vi "textParse.vi"(8 "error in (no error)":errorcluster, 10 "file name":string, 11 "base path":path=path "C:/Users/bryan.lee/Desktop/Specification sheets") -> (0 "error out":errorcluster, 2 "all rows":string[][](array[string]), 3 "appended path":path)   [LabVIEW 2018]
uses:
  <vilib>/Utility/file.llb/Read Delimited Spreadsheet (string).vi
panel:
  out "LED Frequency Max":string
  out "LED Frequency Min":string
  out "LED Frequency (Charge)":string
  out "LED Frequency (Limit)":string
  out "LED Frequency (Foldback)":string
  out "HV Bus Voltage(@10% PWM)":string
  out "HV Bus Tol. Min":string
  out "HV Bus Tol. Max":string
  out "Speed Pot Voltage Low(@85% PWM)":string
  out "Speed Pot Voltage Mid(@85% PWM)":string
  out "Speed Pot Voltage High(@85% PWM)":string
  out "Speed Pot Voltage Tol. Min":string
  out "Speed Pot Voltage Tol. Max":string
  out "Ircomp(@70% PWM)":string
  out "Ircomp Voltage Tol. Min":string
  out "Ircomp Voltage Tol. Max":string
  out "Current Limit(@45% PWM)":string
  out "Sense Voltage Tol. Max":string
  out "Sense Voltage Tol. Min":string
  out "Sense Voltage":string
  out "Allowable Power Interuption":string
  out "Voltage FET Driver Tol. Max":string
  out "Voltage FET Driver Tol. Min":string
  out "Voltage FET Driver":string
  out "Voltage Micro Tol. Max":string
  out "Voltage Micro Tol. Min":string
  out "Voltage Micro":string
  out "Rated Output Current Tol. Max":string
  out "Rated Output Current Tol. Min":string
  out "Rated Output Current":string
  out "Ripple/Noise Tol. Max":string
  out "Ripple/Noise Tol. Min":string
  out "Ripple/Noise":string
  out "Voltage Output Tol. Max":string
  out "Voltage  Output Tol. Min":string
  out "Voltage Output":string
  out "Max Input Current":string
  out "Input Current":string
  out "Input Voltage Tol. Max":string
  out "Input Voltage Tol. Min":string
  out "Input Voltage":string
  out "Vendor Number":string
  out "Vendor Name":string
  out "Firmware":string
  out "Part Number":string
  out "Part Name":string
  # "Global variables"
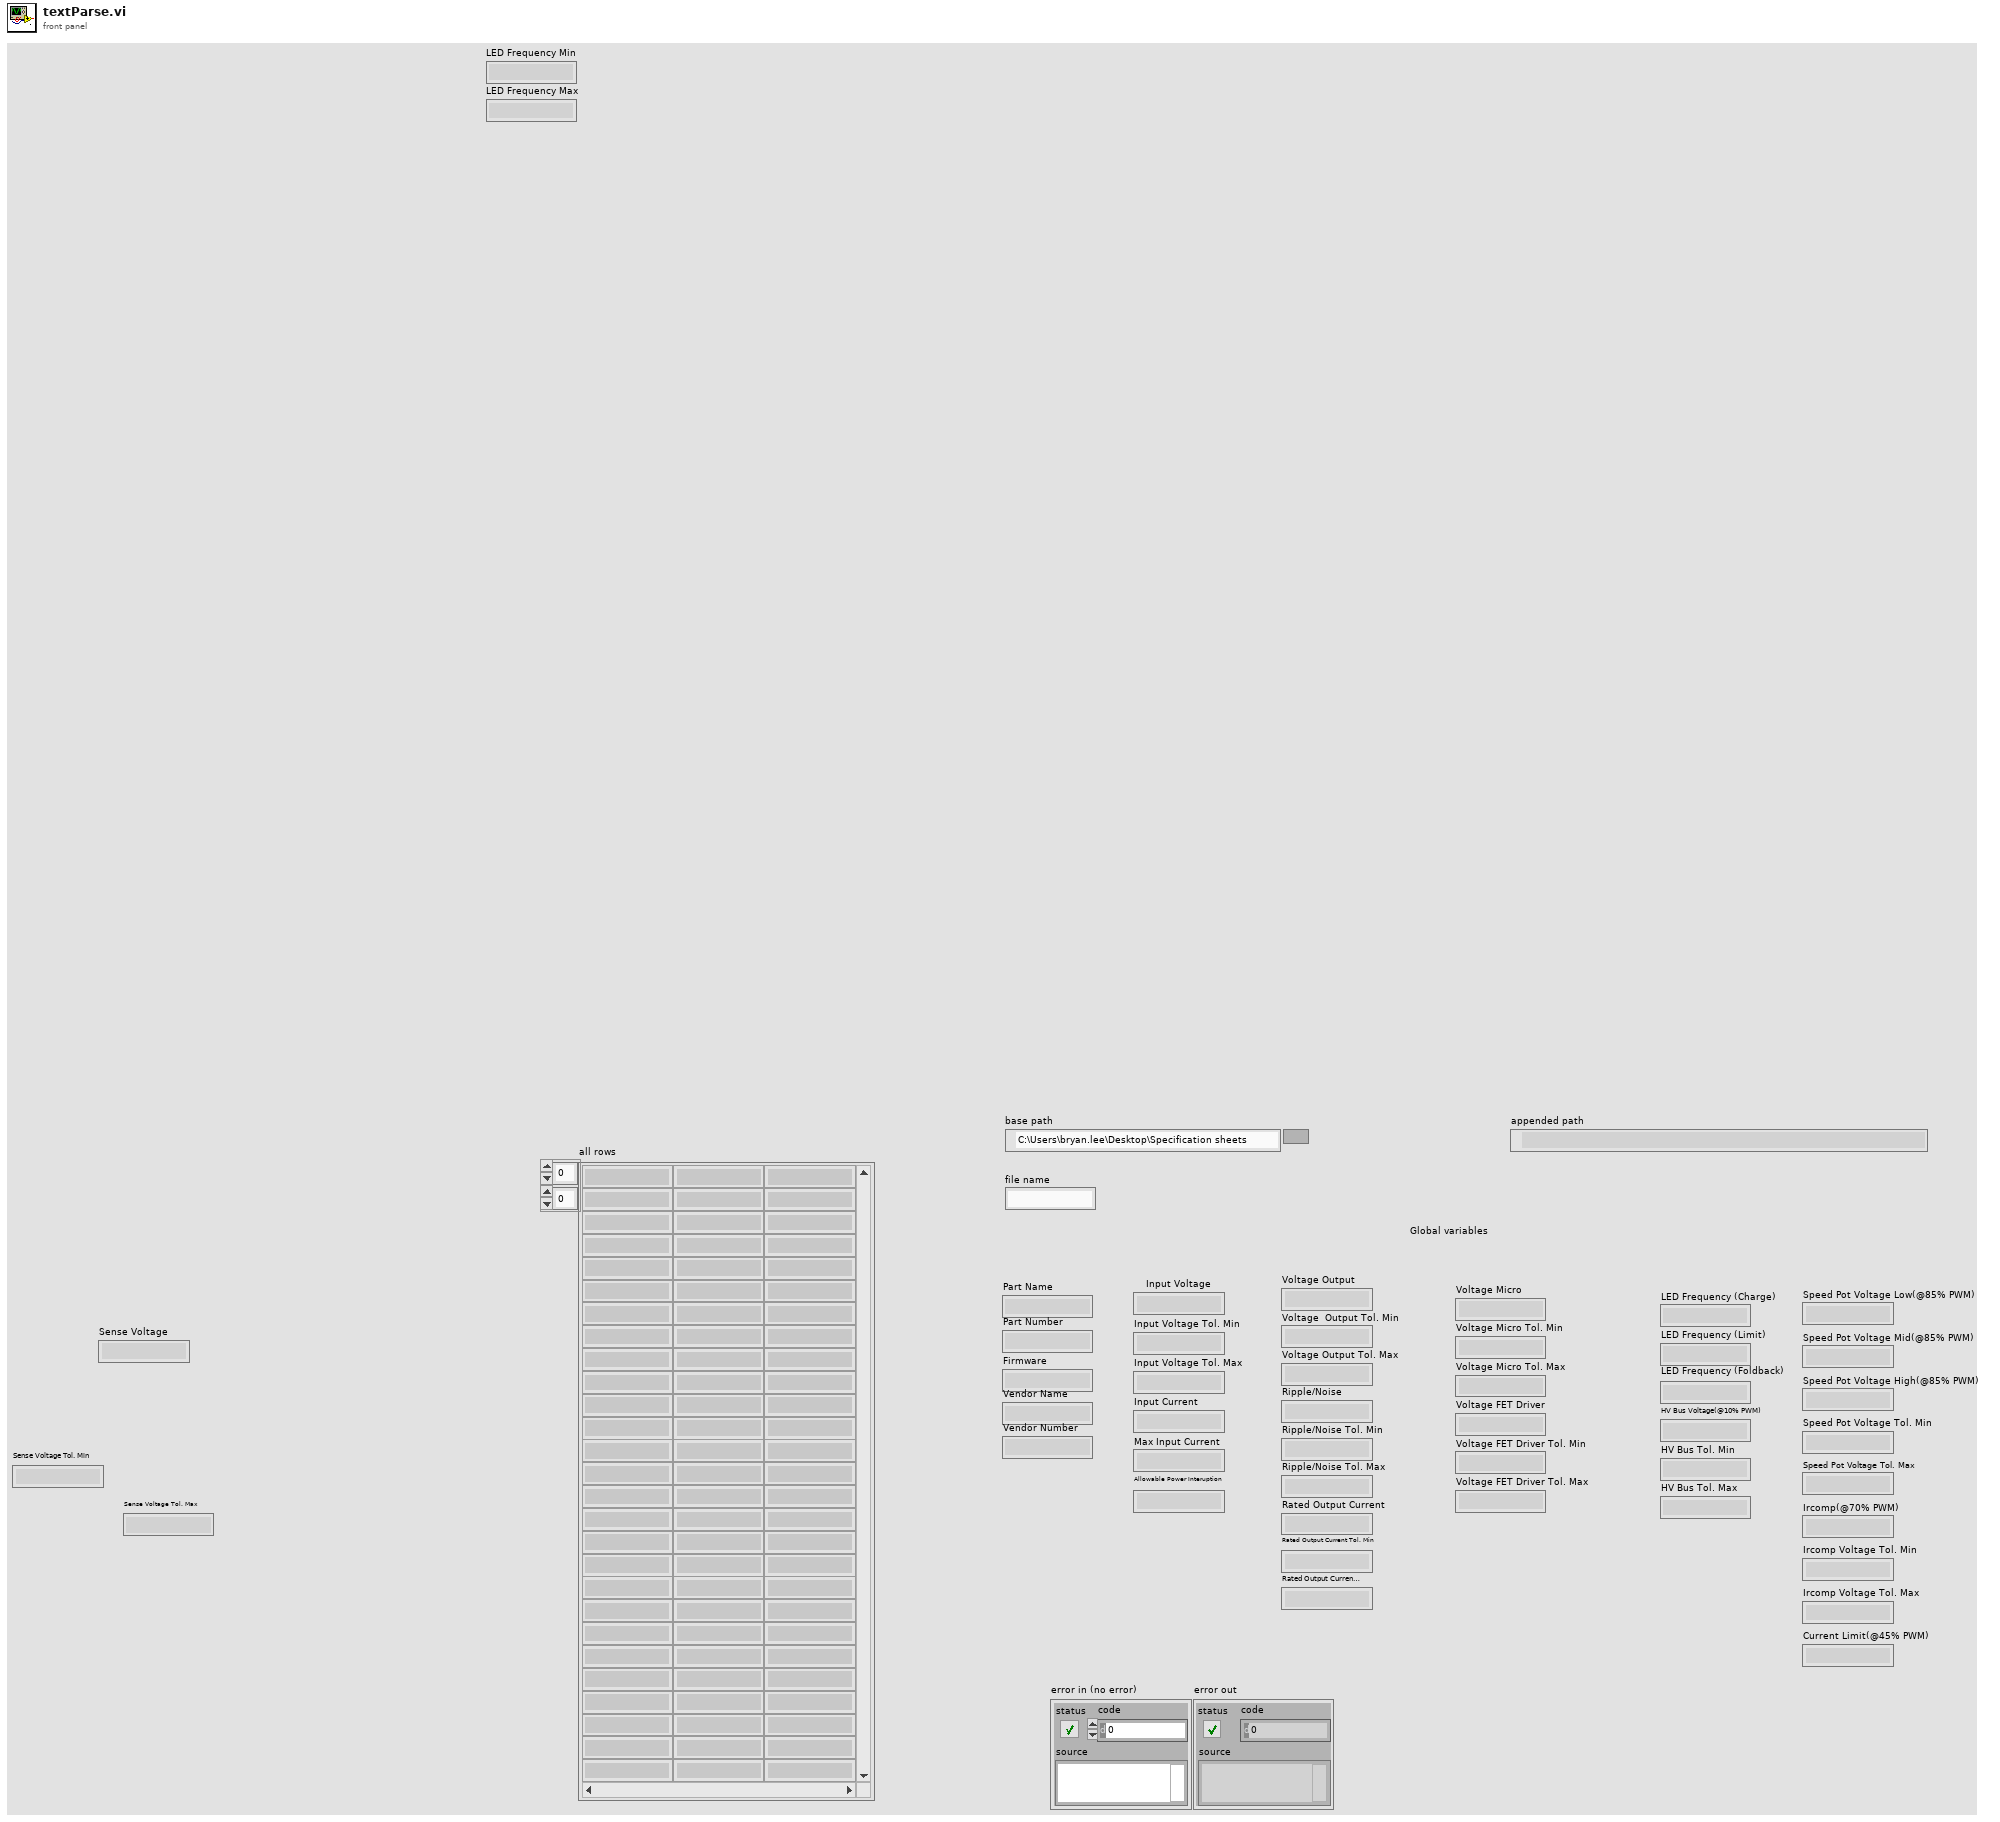
[diagram p1: front panel]
types:
  T1 = enum16{"Main", "In Primary", "Secondary", "Out Primary", "Motor Drive", ""}
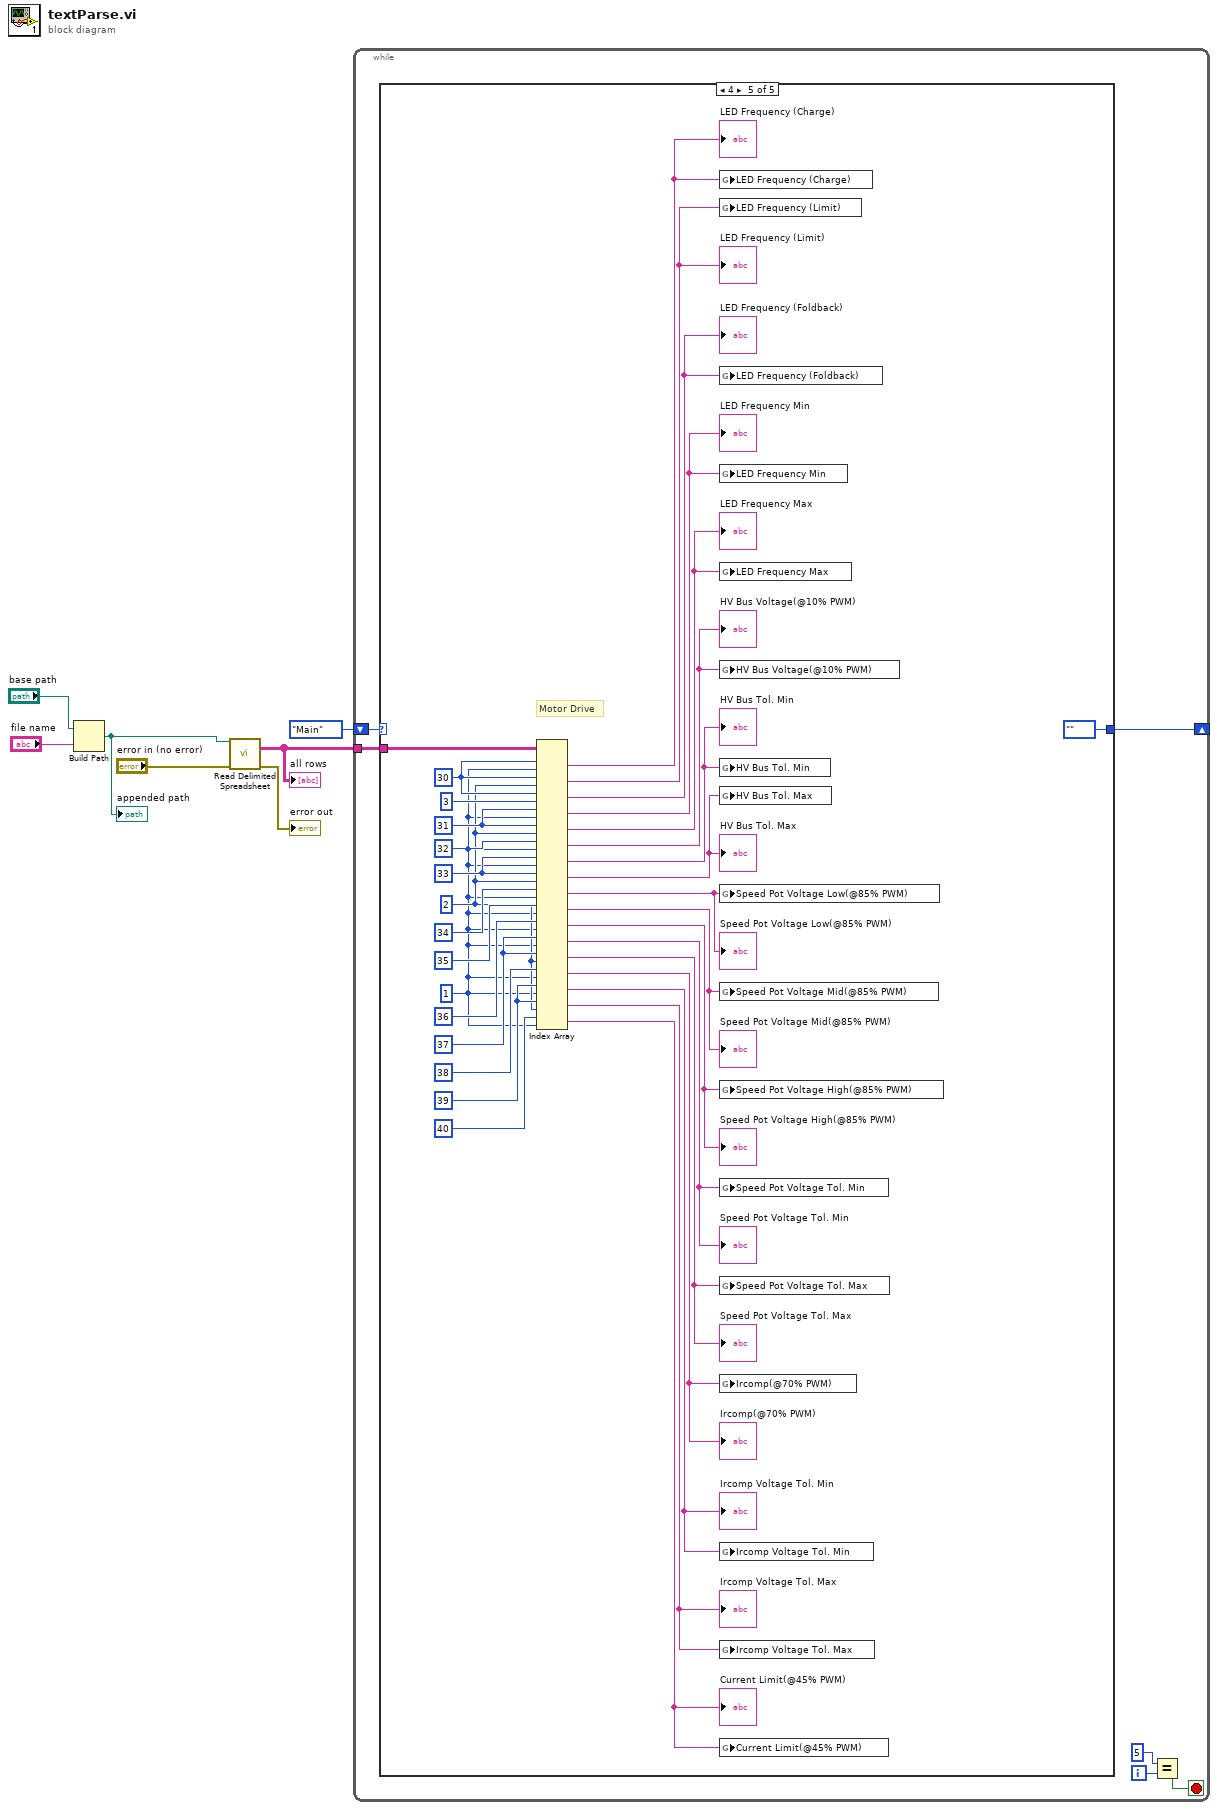
[diagram p0: block diagram]
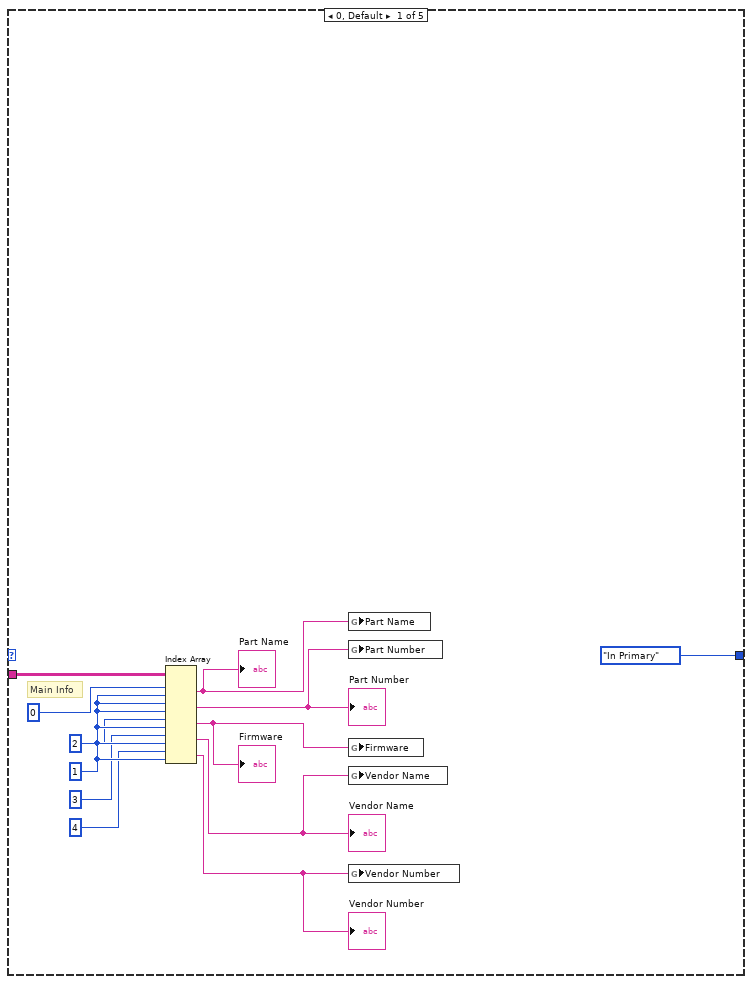
[diagram p2: hidden frame]
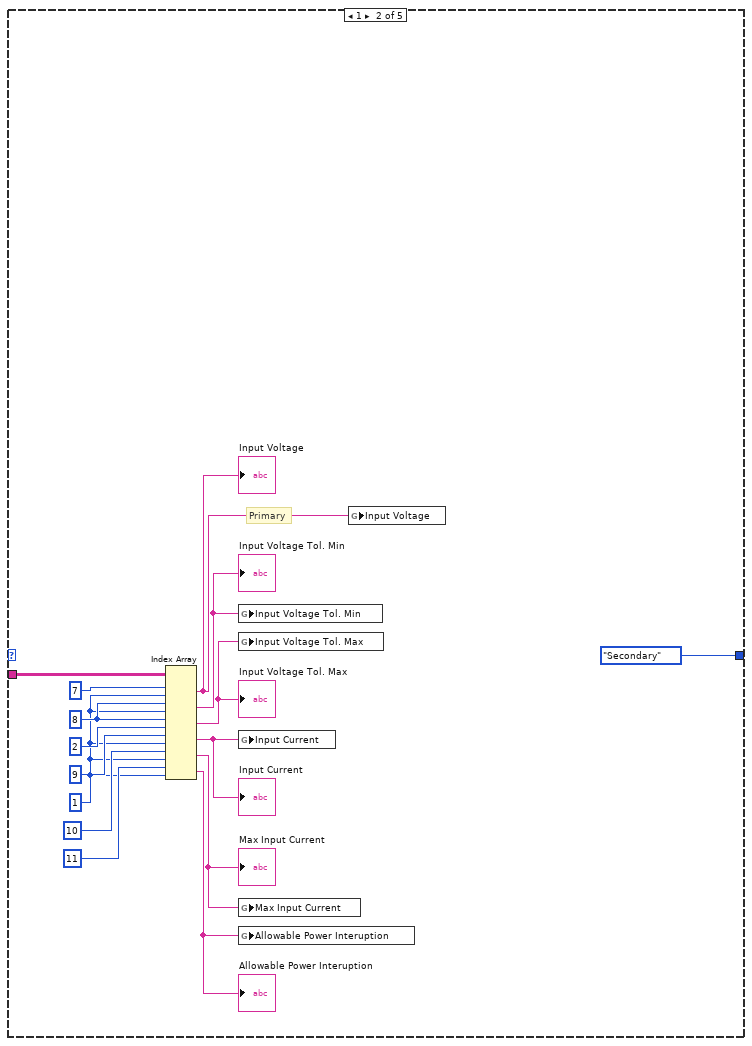
[diagram p3: hidden frame]
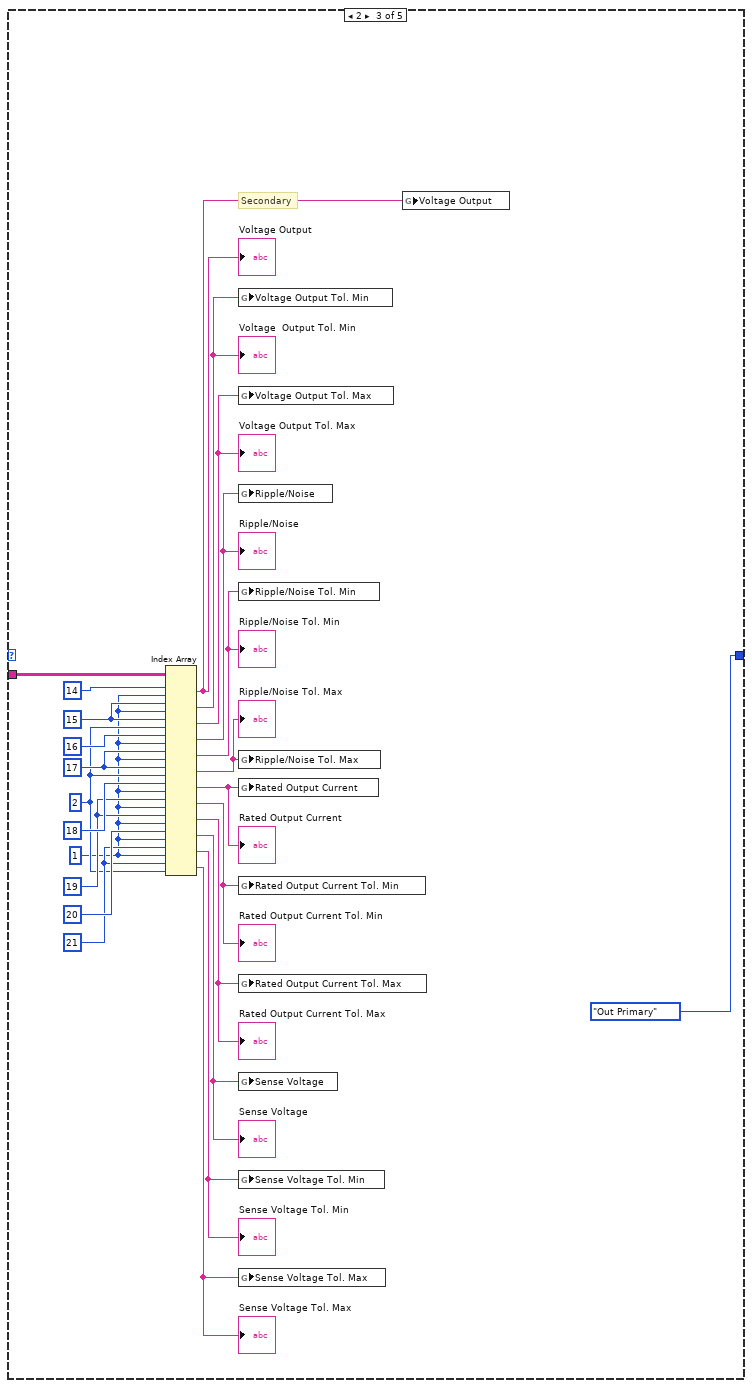
[diagram p4: hidden frame]
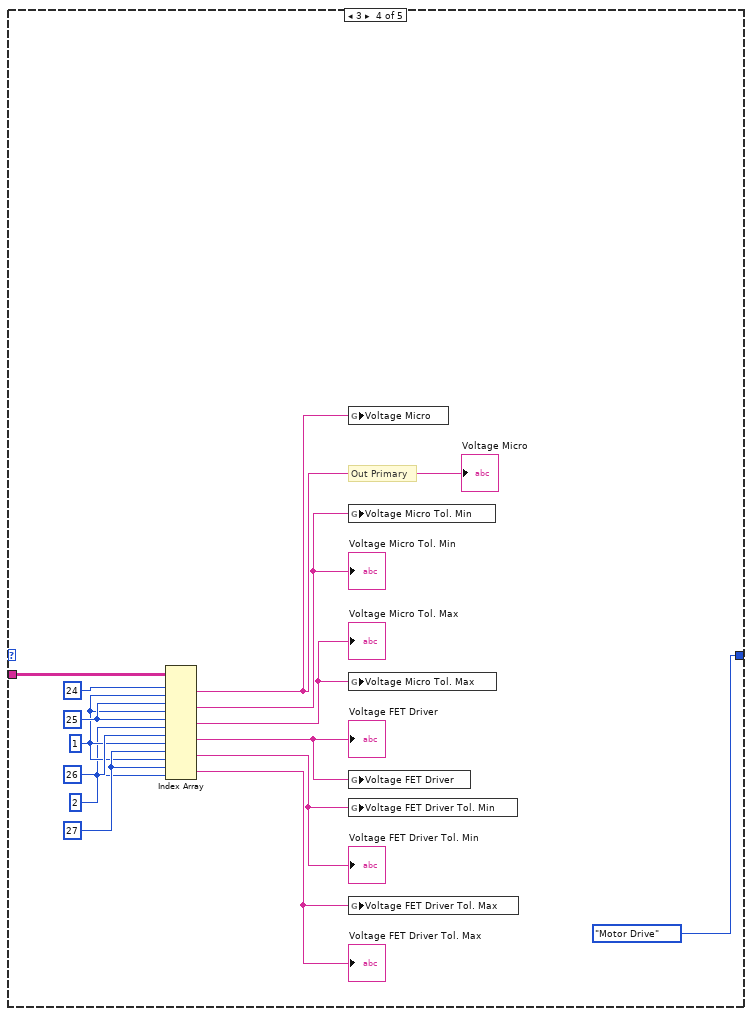
[diagram p5: hidden frame]
diagram:
  n1 = Build Path(base path="base path", name or relative path="file name") -> (appended path=w5:path)
  "appended path" <- w5
  n2 = call-poly <vilib>:"Read Delimited Spreadsheet.vi"("file path (dialog if empty)"=w5, "error in (no error)"="error in (no error)") -> ("all rows"=w2:string[][], "error out"=→"error out":errorcluster)  [unwired: 8 in, 4 out]
  "all rows" <- w2
  n3 = while {
    shift-right: [w12] -> _
    shift-left: T1."Main" -> [w8]
    tunnel: w2 -> [w9]
    i -> [w11]
    stop <- w13 stop-if-true
    n4 = case shown="4" w8 {
      tunnel: w9 -> [w15 w29 w49 w68 w110]
      tunnel: [T1."In Primary" T1."Secondary" T1."Out Primary" T1."Motor Drive" enum16{""}.""] -> w12
      frame 0, Default {
        w19 = 1
        # "Main Info"
        n5 = Index Array(array=w15, index (row) #1=0 ("index (row)"), index (col) #1=w19, index (row) #2=w19, index (col) #2=w19, index (row) #3=2 ("index (row)"), index (col) #3=w19, index (row) #4=3 ("disabled index (row)"), index (col) #4=w19, index (row) #5=4 ("disabled index (row)"), index (col) #5=w19) -> (element #1=w21:string, element #2=w23:string, element #3=w22:string, element #4=w24:string, element #5=w25:string)
        "Part Name" <- w21
        "Part Number" <- w23
        "Firmware" <- w22
        "Vendor Name" <- w24
        "Vendor Number" <- w25
        n6 = global write "Global textParse.vi" "Part Name"(w21) -> ()
        n7 = global write "Global textParse.vi" "Part Number"(w23) -> ()
        n8 = global write "Global textParse.vi" "Firmware"(w22) -> ()
        n9 = global write "Global textParse.vi" "Vendor Name"(w24) -> ()
        n10 = global write "Global textParse.vi" "Vendor Number"(w25) -> ()
      }
      frame 1 {
        w33 = 8
        w27 = 1
        # "Primary"
        n11 = Index Array(array=w29, index (row) #1=7, index (col) #1=w27, index (row) #2=w33, index (col) #2=w27, index (row) #3=w33, index (col) #3=2, index (row) #4=9, index (col) #4=w27, index (row) #5=10, index (col) #5=w27, index (row) #6=11, index (col) #6=w27) -> (element #1=w35:string, element #2=w36:string, element #3=w37:string, element #4=w38:string, element #5=w39:string, element #6=w40:string)
        "Input Voltage" <- w35
        "Input Voltage Tol. Min" <- w36
        "Input Voltage Tol. Max" <- w37
        "Input Current" <- w38
        "Max Input Current" <- w39
        "Allowable Power Interuption" <- w40
        n12 = global write "Global textParse.vi" "Input Voltage Tol. Min"(w36) -> ()
        n13 = global write "Global textParse.vi" "Input Voltage Tol. Max"(w37) -> ()
        n14 = global write "Global textParse.vi" "Input Current"(w38) -> ()
        n15 = global write "Global textParse.vi" "Max Input Current"(w39) -> ()
        n16 = global write "Global textParse.vi" "Allowable Power Interuption"(w40) -> ()
        n17 = global write "Global textParse.vi" "Input Voltage"(w35) -> ()
      }
      frame 2 {
        w47 = 21 ("index (row)")
        w50 = 19 ("index (row)")
        w45 = 1
        w46 = 2
        w52 = 17 ("index (row) 15")
        w54 = 15 ("index (row) 13")
        # "Secondary"
        n18 = Index Array(array=w49, index (row) #1=14 ("index (row) 12"), index (col) #1=w45, index (row) #2=w54, index (col) #2=w45, index (row) #3=w54, index (col) #3=w46, index (row) #4=16 ("index (row) 14"), index (col) #4=w45, index (row) #5=w52, index (col) #5=w45, index (row) #6=w52, index (col) #6=w46, index (row) #7=18 ("index (row) 19"), index (col) #7=w45, index (row) #8=w50, index (col) #8=w45, index (row) #9=w50, index (col) #9=w45, index (row) #10=20 ("index (row)"), index (col) #10=w45, index (row) #11=w47, index (col) #11=w45, index (row) #12=w47, index (col) #12=w46) -> (element #1=w56:string, element #2=w57:string, element #3=w58:string, element #4=w59:string, element #5=w60:string, element #6=w61:string, element #7=w62:string, element #8=w63:string, element #9=w64:string, element #10=w44:string, element #11=w43:string, element #12=w42:string)
        "Voltage Output" <- w56
        "Voltage  Output Tol. Min" <- w57
        "Voltage Output Tol. Max" <- w58
        "Ripple/Noise" <- w59
        "Ripple/Noise Tol. Min" <- w60
        "Ripple/Noise Tol. Max" <- w61
        "Rated Output Current" <- w62
        "Rated Output Current Tol. Min" <- w63
        "Rated Output Current Tol. Max" <- w64
        "Sense Voltage" <- w44
        "Sense Voltage Tol. Min" <- w43
        "Sense Voltage Tol. Max" <- w42
        n19 = global write "Global textParse.vi" "Voltage Output Tol. Min"(w57) -> ()
        n20 = global write "Global textParse.vi" "Voltage Output Tol. Max"(w58) -> ()
        n21 = global write "Global textParse.vi" "Ripple/Noise"(w59) -> ()
        n22 = global write "Global textParse.vi" "Ripple/Noise Tol. Min"(w60) -> ()
        n23 = global write "Global textParse.vi" "Ripple/Noise Tol. Max"(w61) -> ()
        n24 = global write "Global textParse.vi" "Rated Output Current"(w62) -> ()
        n25 = global write "Global textParse.vi" "Rated Output Current Tol. Min"(w63) -> ()
        n26 = global write "Global textParse.vi" "Rated Output Current Tol. Max"(w64) -> ()
        n27 = global write "Global textParse.vi" "Sense Voltage"(w44) -> ()
        n28 = global write "Global textParse.vi" "Sense Voltage Tol. Min"(w43) -> ()
        n29 = global write "Global textParse.vi" "Sense Voltage Tol. Max"(w42) -> ()
        n30 = global write "Global textParse.vi" "Voltage Output"(w56) -> ()
      }
      frame 3 {
        w65 = 2
        w66 = 1
        w69 = 27 ("index (row) 27")
        w71 = 25 ("index (row) 25")
        # "Out Primary"
        n31 = Index Array "Index Array"(array=w68, index (row) #1=24 ("index (row) 24"), index (col) #1=w66, index (row) #2=w71, index (col) #2=w66, index (row) #3=w71, index (col) #3=w65, index (row) #4=26 ("index (row) 26"), index (col) #4=w66, index (row) #5=w69, index (col) #5=w66, index (row) #6=w69, index (col) #6=w65) -> (element #1=w73:string, element #2=w74:string, element #3=w75:string, element #4=w76:string, element #5=w77:string, element #6=w78:string)
        "Voltage Micro" <- w73
        "Voltage Micro Tol. Min" <- w74
        "Voltage Micro Tol. Max" <- w75
        "Voltage FET Driver" <- w76
        "Voltage FET Driver Tol. Min" <- w77
        "Voltage FET Driver Tol. Max" <- w78
        n32 = global write "Global textParse.vi" "Voltage Micro"(w73) -> ()
        n33 = global write "Global textParse.vi" "Voltage Micro Tol. Min"(w74) -> ()
        n34 = global write "Global textParse.vi" "Voltage Micro Tol. Max"(w75) -> ()
        n35 = global write "Global textParse.vi" "Voltage FET Driver"(w76) -> ()
        n36 = global write "Global textParse.vi" "Voltage FET Driver Tol. Min"(w77) -> ()
        n37 = global write "Global textParse.vi" "Voltage FET Driver Tol. Max"(w78) -> ()
      }
      frame 4 {
        w97 = 2
        w96 = 1
        w99 = 39
        w101 = 37
        w105 = 33 ("index (row) 28")
        w107 = 31 ("index (row) 25")
        w108 = 30 ("index (row) 24")
        # "Motor Drive"
        n38 = Index Array "Index Array"(array=w110, index (row) #1=w108, index (col) #1=w96, index (row) #2=w108, index (col) #2=w97, index (row) #3=w108, index (col) #3=3, index (row) #4=w107, index (col) #4=w96, index (row) #5=w107, index (col) #5=w97, index (row) #6=32 ("index (row) 26"), index (col) #6=w96, index (row) #7=w105, index (col) #7=w96, index (row) #8=w105, index (col) #8=w97, index (row) #9=34 ("index (row) 29"), index (col) #9=w96, index (row) #10=35, index (col) #10=w96, index (row) #11=36 ("index (row) 30"), index (col) #11=w96, index (row) #12=w101, index (col) #12=w96, index (row) #13=w101, index (col) #13=w97, index (row) #14=38, index (col) #14=w96, index (row) #15=w99, index (col) #15=w96, index (row) #16=w99, index (col) #16=w97, index (row) #17=40, index (col) #17=w96) -> (element #1=w95:string, element #2=w94:string, element #3=w93:string, element #4=w92:string, element #5=w91:string, element #6=w90:string, element #7=w89:string, element #8=w88:string, element #9=w87:string, element #10=w86:string, element #11=w85:string, element #12=w84:string, element #13=w83:string, element #14=w82:string, element #15=w81:string, element #16=w80:string, element #17=w79:string)
        "LED Frequency (Charge)" <- w95
        "LED Frequency (Limit)" <- w94
        "LED Frequency (Foldback)" <- w93
        "HV Bus Voltage(@10% PWM)" <- w90
        "HV Bus Tol. Min" <- w89
        "HV Bus Tol. Max" <- w88
        "Speed Pot Voltage Low(@85% PWM)" <- w87
        "Speed Pot Voltage Mid(@85% PWM)" <- w86
        "Speed Pot Voltage High(@85% PWM)" <- w85
        "Speed Pot Voltage Tol. Min" <- w84
        "Speed Pot Voltage Tol. Max" <- w83
        "Ircomp(@70% PWM)" <- w82
        "Ircomp Voltage Tol. Min" <- w81
        "Ircomp Voltage Tol. Max" <- w80
        "Current Limit(@45% PWM)" <- w79
        "LED Frequency Min" <- w92
        "LED Frequency Max" <- w91
        n39 = global write "Global textParse.vi" "LED Frequency (Charge)"(w95) -> ()
        n40 = global write "Global textParse.vi" "LED Frequency (Limit)"(w94) -> ()
        n41 = global write "Global textParse.vi" "LED Frequency (Foldback)"(w93) -> ()
        n42 = global write "Global textParse.vi" "LED Frequency Min"(w92) -> ()
        n43 = global write "Global textParse.vi" "LED Frequency Max"(w91) -> ()
        n44 = global write "Global textParse.vi" "HV Bus Voltage(@10% PWM)"(w90) -> ()
        n45 = global write "Global textParse.vi" "HV Bus Tol. Min"(w89) -> ()
        n46 = global write "Global textParse.vi" "HV Bus Tol. Max"(w88) -> ()
        n47 = global write "Global textParse.vi" "Speed Pot Voltage Low(@85% PWM)"(w87) -> ()
        n48 = global write "Global textParse.vi" "Speed Pot Voltage Mid(@85% PWM)"(w86) -> ()
        n49 = global write "Global textParse.vi" "Speed Pot Voltage High(@85% PWM)"(w85) -> ()
        n50 = global write "Global textParse.vi" "Speed Pot Voltage Tol. Min"(w84) -> ()
        n51 = global write "Global textParse.vi" "Speed Pot Voltage Tol. Max"(w83) -> ()
        n52 = global write "Global textParse.vi" "Ircomp(@70% PWM)"(w82) -> ()
        n53 = global write "Global textParse.vi" "Ircomp Voltage Tol. Min"(w81) -> ()
        n54 = global write "Global textParse.vi" "Ircomp Voltage Tol. Max"(w80) -> ()
        n55 = global write "Global textParse.vi" "Current Limit(@45% PWM)"(w79) -> ()
      }
    }
    n56 = Equal?(x=5, y=w11) -> (x = y?=w13:bool)
  }
